vi "StimGenRun.vi"(3 "error in":errorcluster, 5 "stimulus specifier":T1) -> (0 "error out":errorcluster, 1 "timing uncertainty (s)":dbl, 2 "stimulus specifier":T1)   [LabVIEW 2014]
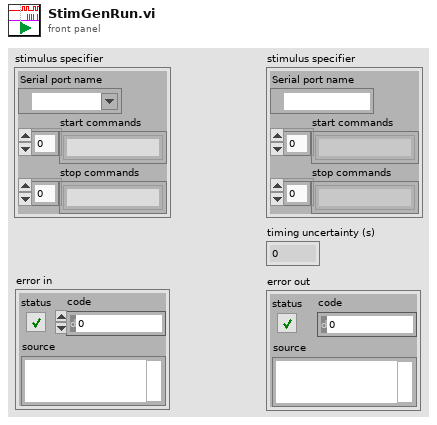
[diagram p1: front panel]
types:
  T1 = cluster{"Serial port name":refnum<visa-resource-name>, "start commands":string[], "stop commands":string[]}
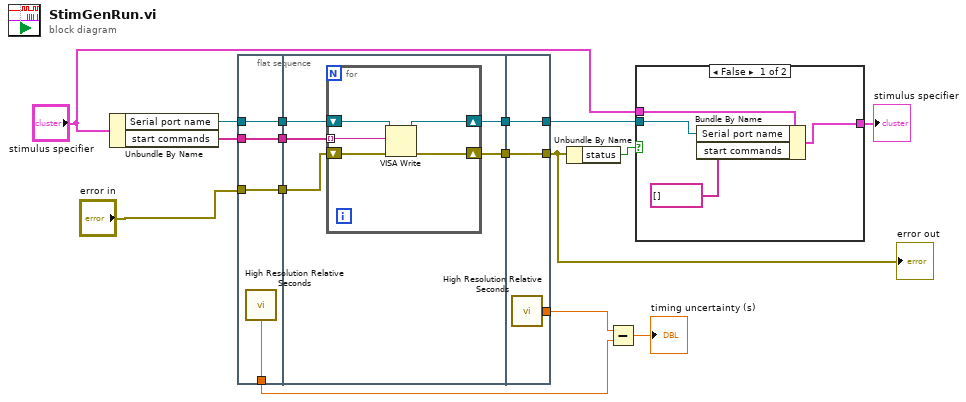
[diagram p0: block diagram]
diagram:
  n1 = Unbundle By Name("stimulus specifier") -> ("Serial port name"=w15:refnum<visa-resource-name>, "start commands"=w16:string[])
  n2 = flat-sequence {
    tunnel: "error in" -> [w18]
    tunnel: w15 -> [w19]
    tunnel: w16 -> [w20]
    tunnel: [w20] -> w8
    tunnel: [w19] -> w7
    tunnel: [w18] -> w6
    tunnel: [w17] -> w4
    tunnel: [w22] -> w10
    tunnel: [w21] -> w9
    tunnel: w8 -> [w25]
    tunnel: w7 -> [w24]
    tunnel: w6 -> [w23]
    tunnel: [w32] -> w11
    tunnel: [w33] -> w14
    tunnel: w10 -> [w33]
    tunnel: w9 -> [w32]
    tunnel: [w31] -> w5
    frame #0 {
      n3 = call <vilib>:"High Resolution Relative Seconds.vi"() -> ("relative seconds"=w17:dbl)
    }
    frame #1 {
      n4 = for {
        tunnel: w25 -> [w29] mode=indexing
        shift-right: [w27] -> w22
        shift-left: w23 -> [w28]
        shift-right: [w26] -> w21
        shift-left: w24 -> [w30]
        n5 = VISA Write(VISA resource name=w30, write buffer=w29, error in (no error)=w28) -> (VISA resource name out=w26:refnum<visa-resource-name>, error out=w27:errorcluster)  [unwired: 1 out]
      }
    }
    frame #2 {
      n6 = call <vilib>:"High Resolution Relative Seconds.vi"() -> ("relative seconds"=w31:dbl)
    }
  }
  n7 = Unbundle By Name(w14) -> ("status"=w13:bool)
  n8 = Subtract(x=w5, y=w4) -> (x-y=→"timing uncertainty (s)":dbl)
  n9 = case shown="False" w13 {
    tunnel: "stimulus specifier" -> [w37 w38]
    tunnel: [w36 w38] -> w3
    tunnel: w11 -> [w35 _]
    frame False {
      n10 = Bundle By Name(cluster=w37, "Serial port name"=w35, "start commands"=string[] []) -> (w36:T1)
    }
    frame True {
    }
  }
  "stimulus specifier" <- w3
  "error out" <- w14
